vi "setFPGAReference.vi"(10 "FPGAReference":refnum<k20>, 11 "ModbusFactory in":refnum<class "ModbusFactory.lvclass">) -> (3 "ModbusFactory out":refnum<class "ModbusFactory.lvclass">)   [LabVIEW 2016, in "ModbusFactory.lvclass"]
uses:
  ModbusFactory.lvclass
  ModbusFactory.lvclass/ModbusFactory.ctl
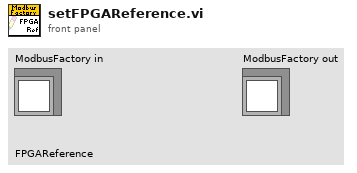
[diagram p1: front panel]
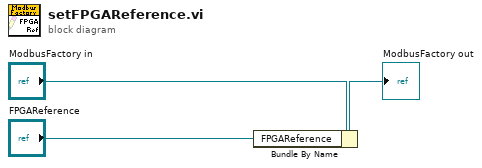
[diagram p0: block diagram]
diagram:
  n1 = Bundle By Name(cluster="ModbusFactory in", "FPGAReference"="FPGAReference") -> (→"ModbusFactory out":refnum<class "ModbusFactory.lvclass">)
